vi "Read_RD_Ch_header.vi"(0 "Raw data file":path) -> (1 "Ch Name Out":string[](array[string]), 2 "Ch Values":string[](array[string]), 3 "Ch string":string, 4 "Comments":string[](array[string]))   [LabVIEW 2011]
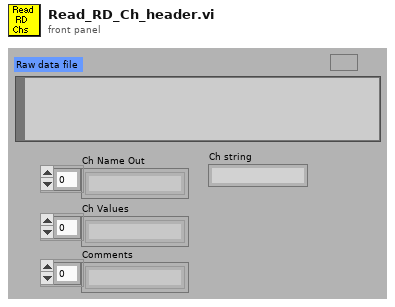
[diagram p1: front panel]
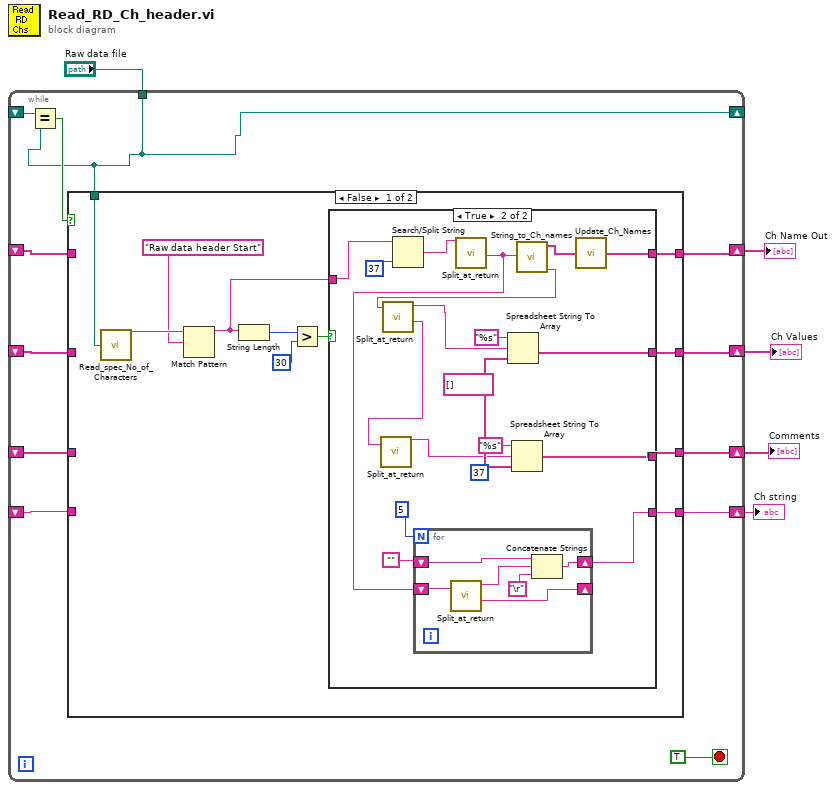
[diagram p0: block diagram]
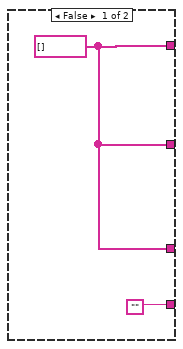
[diagram p2: hidden frame]
diagram:
  n1 = while {
    shift-right: [w8] -> _
    shift-left: _ -> [w9]
    shift-right: [w16] -> w3
    shift-left: _ -> [w13]
    shift-right: [w15] -> w5
    shift-left: _ -> [w12]
    shift-right: [w14] -> w4
    shift-left: _ -> [w11]
    tunnel: "Raw data file" -> [w8]
    shift-right: [w7] -> w1
    shift-left: _ -> [w6]
    stop <- TRUE stop-if-true
    n2 = Equal?(x=w9, y=w8) -> (x = y?=w17:bool)
    n3 = case shown="False" w17 {
      tunnel: [w22 w58] -> w16
      tunnel: [w21 w57] -> w15
      tunnel: [w20 w56] -> w14
      tunnel: w13 -> [_ w58]
      tunnel: w12 -> [_ w57]
      tunnel: w11 -> [_ w56]
      tunnel: w8 -> [w19 _]
      tunnel: [w18 w55] -> w7
      tunnel: w6 -> [_ w55]
      frame False {
        n4 = call "Read_spec_No_of_Characters.vi"("Filename"=w19) -> ("character string"=w28:string)  [unwired: 1 out]
        n5 = Match Pattern(string=w28, regular expression="Raw data header Start") -> (before substring=w24:string)  [unwired: 4 out]
        n6 = String Length(string=w24) -> (length=w23:i32)
        n7 = Greater?(x=w23, y=30) -> (0:w25:bool)
        n8 = case shown="True" w25 {
          tunnel: w24 -> [_ w37]
          tunnel: [w30 w35] -> w22
          tunnel: [w30 w41] -> w21
          tunnel: [w30 w40] -> w20
          tunnel: ["" w31] -> w18
          frame False {
            w30 = string[] [] ("Ch Name Out")
          }
          frame True {
            (unwired) 37 ("y")
            w43 = string[] [] ("Channel Values")
            n9 = Search/Split String(string=w37, offset (0)=37 ("y")) -> (match + rest of string=w38:string)  [unwired: 3 out]
            n10 = call "Split_at_return.vi"("String"=w38) -> ("after substring"=w33:string)  [unwired: 1 in, 3 out]
            n11 = for {
              N: 5 -> [_]
              shift-right: [w52] -> w31
              shift-left: "" -> [w54]
              shift-right: [w50] -> _
              shift-left: w33 -> [w51]
              n12 = call "Split_at_return.vi"("String"=w51) -> ("before substring"=w53:string, "after substring"=w50:string)  [unwired: 1 in, 2 out]
              n13 = Concatenate Strings(w54, w53, "\r") -> (w52:string)
            }
            n14 = call "String_to_Ch_names.vi"("Spreadsheet string"=w33) -> ("Ch names"=w36:string[], "String After names"=w47:string)  [unwired: 2 out]
            n15 = call "Split_at_return.vi"("String"=w47) -> ("before substring"=w46:string, "after substring"=w45:string)  [unwired: 1 in, 2 out]
            n16 = call "Split_at_return.vi"("String"=w45) -> ("before substring"=w42:string)  [unwired: 1 in, 3 out]
            n17 = Spreadsheet String To Array(format string="%s", spreadsheet string=w46, array type (2D Dbl)=w43) -> (array=w41:string[])  [unwired: 1 out]
            n18 = Spreadsheet String To Array(format string="%s", spreadsheet string=w42, array type (2D Dbl)=w43) -> (array=w40:string[])  [unwired: 1 out]
            n19 = call "Update_Ch_Names.vi"("Ch Name in"=w36) -> ("Ch Name Out"=w35:string[])
          }
        }
      }
      frame True {
      }
    }
  }
  "Ch Name Out" <- w3
  "Ch Values" <- w5
  "Comments" <- w4
  "Ch string" <- w1
